vi "rep_cap_compose_cmd.vi"(5 "Repeated Capability":string, 7 "Attribute":T1={"Identifier"="", "Descriptive Name"="", "Data Type"=enum."Integer 32", "Command"="", "Access"=enum."Read/Write", "Range Table"="", "Read Callback"="", "Write Callback"="", "Supported Models"="", "Instrument Options"="", "Index"=0, "OPC Wait"=FALSE, "No Status Check"=FALSE, "Cache Only"=FALSE}, 8 "error in":errorcluster caption="error in (no error)", 11 "VISA resource name":refnum<visa-resource-name>) -> (0 "error out":errorcluster, 2 "Command out":string, 3 "VISA resource name out":refnum<visa-resource-name>)   [LabVIEW 2022 SP3, in "hmp4000_rsidr_core.lvlib"]
uses:
  hmp4000_rsidr_core.lvlib
  type_Attribute.ctl
  type_Attribute_Data_Type.ctl
  type_ReadWriteAccess.ctl
  type_AdditionalFlag_Bits.ctl
  _type_Operation_Fgv_RepCap.ctl
  type_Error_Codes.ctl
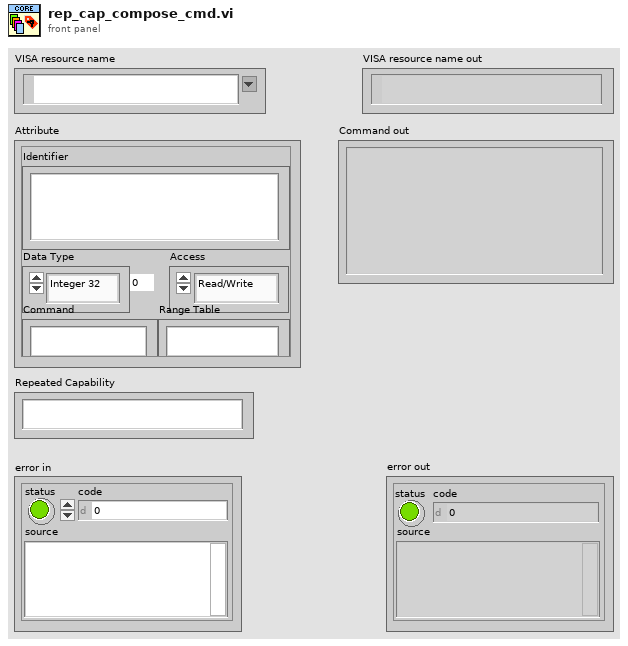
[diagram p1: front panel]
types:
  T1 = typedef "hmp4000_rsidr_core.lvlib/type_Attribute.ctl" = cluster{"Identifier":string, "Descriptive Name":string, "Data Type":T2, "Command":string, "Access":T3, "Range Table":string, "Read Callback":string, "Write Callback":string, "Supported Models":string, "Instrument Options":string, "Index":i32, "OPC Wait":bool, "No Status Check":bool, "Cache Only":bool}
  T2 = typedef "hmp4000_rsidr_core.lvlib/type_Attribute_Data_Type.ctl" = enum16{"Integer 32", "Double", "String", "Boolean", "None", "Integer 64", "RawString"}
  T3 = typedef "hmp4000_rsidr_core.lvlib/type_ReadWriteAccess.ctl" = enum16{"Read Only", "Write Only", "Read/Write"}
  T4 = typedef "hmp4000_rsidr_core.lvlib/type_AdditionalFlag_Bits.ctl" = enum16{"Send LF after Bin Block", "Junk read with io_clear_buffers.vi", "io_clear_buffers: viClear()", "io_clear_buffers: viFlush()", "<NotUsed1>", "Allow Dbl & Int Bin/Ascii read", "*OPC? in check_instrument_error.vi", "<NotUsed2>", "Smart Enum Matching", "Less Strict RepCaps check", "AssureResponseEndWithLF"}
  T5 = typedef "hmp4000_rsidr_core.lvlib/_type_Operation_Fgv_RepCap.ctl" = enum16{"Initialize", "Get Cmd Value", "Reset Rep Cap", "Add Rep Cap", "Remove Rep Cap", "Get Rep Cap ID range", "Get Count", "Clear", "Find Name from NameID", "Get First NameID"}
  T6 = typedef "hmp4000_rsidr_core.lvlib/type_Error_Codes.ctl" = enum16{"No_error", "VISA_err_ResourceNotFound", "VISA_err_Timeout", "VISA_warn_MoreDataAvailable", "RS_err_MissingCallback", "RS_err_InvalidAttribute", "RS_err_InvalidValue", "RS_err_UnknownResource", "RS_err_AlreadyInitialized", "RS_err_InstrumentStatus", "RS_err_BadRepCapName", "RS_err_TypesMismatch", "RS_err_ValueNotSupported", "RS_err_InvalidRngTable", "RS_err_IDqueryFail", "RS_err_UnexpResponse", "VISA_warn_ConfigNotLoaded", "RS_err_AttributeNotReadable", "RS_err_AttributeNotWritable", "RS_err_InstrumentType", "RS_err_InstrumentOption", "VISA_err_InvalidSize", "RS_err_ReliabilityIndicator", "VISA_warn_UnknownStatus", "VISA_warn_TermCharRead", "VISA_err_IO_error", "RS_err_FunctionNotSupported", "VISA_warn_QueueEmpty"}
  T7 = typedef "hmp4000_rsidr_core.lvlib/type_Session_Data.ctl" = cluster{"IDN string":string, "Instrument FW":string, "Instr type":string, "Instr type for err. msg.":string, "Installed Options":string[], "Ignore Error Messages":string, "Logging params":variant, "OPC Timeout":i32, "VISA Timeout":i32, "STB Poll VISA Timeout":i32, "Additional Flags":i32, "Wait Before Read":i32, "Wait Before Write":i32, "Option String Flags":i32, "IO Segment Size":i64, "VISA Access Mode":T8, "Interface Type":T9, "OPC Wait Mode":T10, "Bin Float Number  Format":T11, "Bin Integer Number Format":T12, "Simulate":bool, "VXIcapable":bool, "Duplicate Session":bool, "Add LF to Write":bool, "Logging":bool, "Fast Sweep":bool, "Query Instrument Status":bool, "Check Range":bool, "Check Options":bool}
  T8 = typedef "hmp4000_rsidr_core.lvlib/type_VisaAccessMode.ctl" = u16
  T9 = typedef "hmp4000_rsidr_core.lvlib/type_InterfaceType.ctl" = enum16{"Unknown", "GPIB", "VXI", "GPIB_VXI", "ASRL", "PXI", "TCPIP", "USB", "SOCKET"}
  T10 = typedef "hmp4000_rsidr_core.lvlib/type_OPC_Wait_Mode.ctl" = enum16{"STBpolling", "STBpollingSlow", "STBpollingSuperSlow", "ServiceRequest", "OPCquery"}
  T11 = typedef "hmp4000_rsidr_core.lvlib/type_Binary_Float_Number_Format.ctl" = enum16{"Float_4_Bytes_Swapped", "Float_4_Bytes", "Double_8_Bytes_Swapped", "Double_8_Bytes"}
  T12 = typedef "hmp4000_rsidr_core.lvlib/type_Binary_Integer_Number_Format.ctl" = enum16{"Int32_4_Bytes_Swapped", "Int32_4 Bytes", "Int16_2_Bytes_Swapped", "Int16_2_Bytes"}
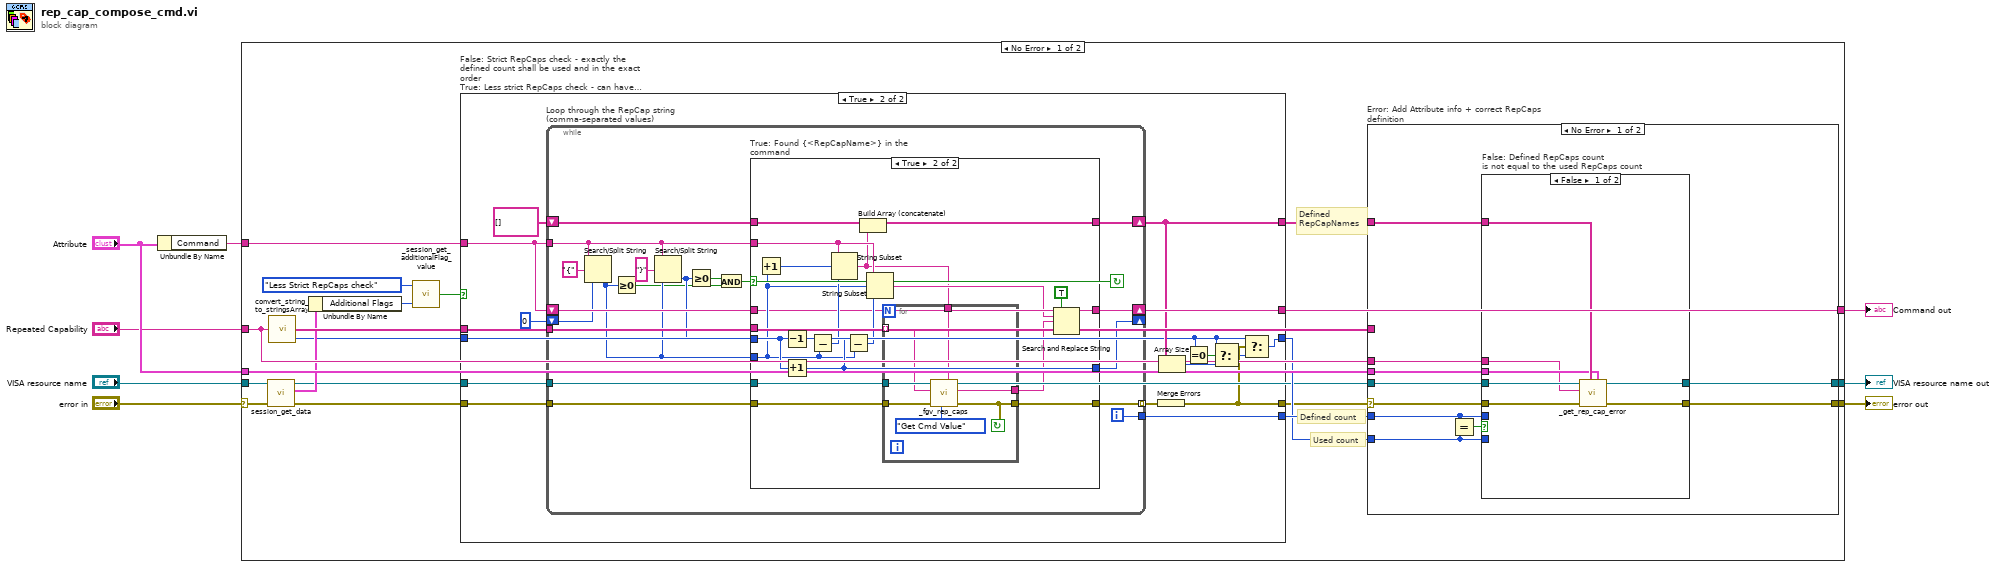
[diagram p0: block diagram]
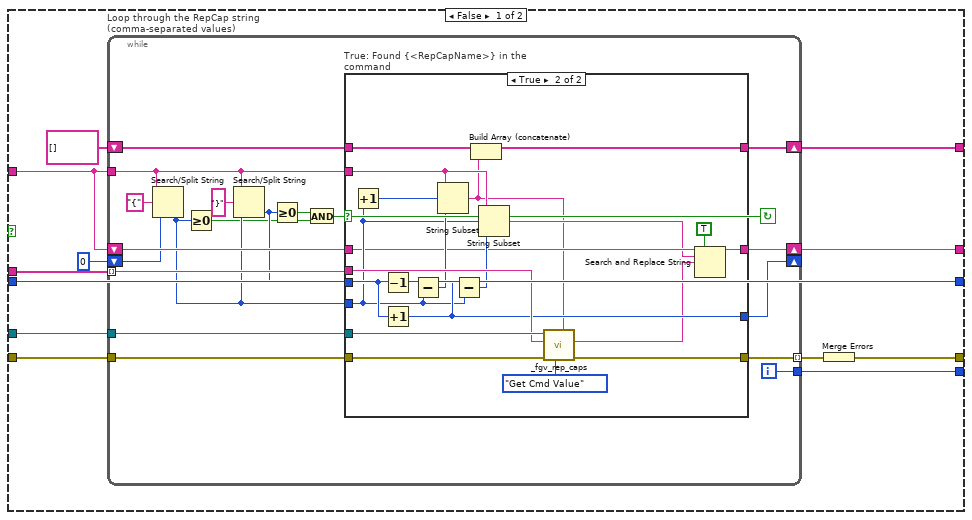
[diagram p2: hidden frame]
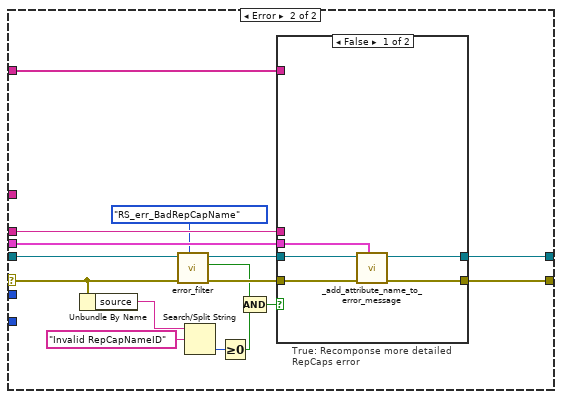
[diagram p6: hidden frame]
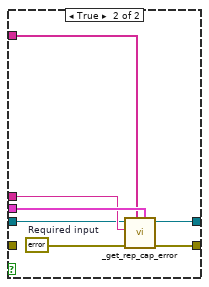
[diagram p7: hidden frame]
diagram:
  n1 = Unbundle By Name("Attribute") -> ("Command"=w1:string)
  n2 = case shown="No Error" "error in" {
    selector: "error in" -> [w19 w198]
    tunnel: "Repeated Capability" -> [w22 _]
    tunnel: [w28 w197] -> w8
    tunnel: [w25 w198] -> w7
    tunnel: w1 -> [w27 w197]
    tunnel: "VISA resource name" -> [w18 w196]
    tunnel: "Attribute" -> [w24 _]
    tunnel: [w21 w196] -> w6
    frame No Error {
      # "Defined count"
      # "Used count"
      # "Defined\nRepCapNames"
      n3 = call "session_get_data.vi"("error in"=w19, "VISA resource name"=w18) -> ("error out"=w17:errorcluster, "Session User Data out"=w16:T7, "VISA resource name out"=w10:refnum<visa-resource-name>)  [unwired: 6 in, 1 out]
      n4 = call "convert_string_to_stringsArray.vi"("String in"=w22) -> ("string array size out"=w13:i32, "string array out"=w20:string[])  [unwired: 3 in]
      n5 = Unbundle By Name(w16) -> ("Additional Flags"=w15:i32)
      n6 = call "_session_get_additionalFlag_value.vi"("AdditionalFlags value in"=w15, "AdditionalFlag bit"=type_AdditionalFlag_Bits."Less Strict RepCaps check") -> ("AdditionalFlag bit value out"=w9:bool)  [unwired: 3 in]
      n7 = case "False: Strict RepCaps check - exactly the defined count shall be used and in the exact order\nTrue: Less strict RepCaps check - can have more repcaps and they can be in random order" shown="True" w9 {
        tunnel: [w40 w99] -> w28
        tunnel: w17 -> [w39 w98]
        tunnel: w27 -> [w38 w97]
        tunnel: [w36 w95] -> w26
        tunnel: [w34 w91] -> w23
        tunnel: [w29 w89] -> w11
        tunnel: w10 -> [w33 w93]
        tunnel: w20 -> [w32 w92]
        tunnel: w13 -> [w31 w85]
        tunnel: [w31 w88] -> w12
        frame False {
          n8 = while "Loop through the RepCap string (comma-separated values)" {
            shift-right: [w59] -> w40
            shift-left: w38 -> [w58]
            tunnel: w33 -> [w56]
            tunnel: w32 -> [w55] mode=indexing
            tunnel: w38 -> [w52]
            shift-right: [w53] -> _
            shift-left: 0 -> [w42]
            tunnel: w39 -> [w57]
            tunnel: [w50] -> w30 mode=indexing
            tunnel: [w45] -> w36
            shift-right: [w43] -> w34
            shift-left: string[] [] -> [w44]
            i -> [w45]
            stop <- w41 continue-if-true
            n9 = Search/Split String(string=w52, search string/char (-)="{", offset (0)=w42) -> (offset of match=w51:i32)  [unwired: 2 out]
            n10 = Greater Or Equal To 0?(x=w51) -> (x >= 0?=w47:bool)
            n11 = Search/Split String(string=w52, search string/char (-)="}", offset (0)=w51) -> (offset of match=w48:i32)  [unwired: 2 out]
            n12 = Greater Or Equal To 0?(x=w48) -> (x >= 0?=w46:bool)
            n13 = And(x=w46, y=w47) -> (x .and. y?=w41:bool)
            n14 = case "True: Found {<RepCapName>} in the command" shown="True" w41 {
              tunnel: w58 -> [w62 w72]
              tunnel: [w62 w70] -> w59
              tunnel: [w61 w71] -> w50
              tunnel: w57 -> [w61 w82]
              tunnel: w56 -> [_ w83]
              tunnel: w55 -> [_ w81]
              tunnel: w48 -> [_ w76]
              tunnel: w51 -> [_ w73]
              tunnel: [_ w75] -> w53
              tunnel: w52 -> [_ w77]
              tunnel: w44 -> [w60 w68]
              tunnel: [w60 w67] -> w43
              frame False {
              }
              frame True {
                n15 = Increment(x=w73) -> (x+1=w80:i32)
                n16 = Decrement(x=w76) -> (x-1=w79:i32)
                n17 = Increment(x=w76) -> (x+1=w75:i32)
                n18 = Subtract(x=w79, y=w73) -> (x-y=w78:i32)
                n19 = String Subset(string=w77, offset (0)=w80, length (rest)=w78) -> (substring=w66:string)
                n20 = Subtract(x=w75, y=w73) -> (x-y=w74:i32)
                n21 = Build Array (concatenate)(w68, w66) -> (w67:string[])
                n22 = String Subset(string=w77, offset (0)=w73, length (rest)=w74) -> (substring=w69:string)
                n23 = call "_fgv_rep_caps.vi"("RepCapName in (\"\")"=w66, "Operation"=_type_Operation_Fgv_RepCap."Get Cmd Value", "error in"=w82, "RepCapNameID in (\"\")"=w81, "VISA resource name"=w83) -> ("error out"=w71:errorcluster, "CmdValue out"=w65:string)  [unwired: 3 in, 2 out]
                n24 = Search and Replace String(replace all?=TRUE ("replace all? (F)"), input string=w72, search string=w69, replace string=w65) -> (result string=w70:string)  [unwired: 4 in, 3 out]
              }
            }
          }
          n25 = Merge Errors(w30) -> (w29:errorcluster)
        }
        frame True {
          n26 = while "Loop through the RepCap string (comma-separated values)" {
            shift-right: [w118] -> w99
            shift-left: w97 -> [w117]
            tunnel: w93 -> [w115]
            tunnel: w92 -> [w114]
            tunnel: w97 -> [w111]
            shift-right: [w112] -> _
            shift-left: 0 -> [w101]
            tunnel: w98 -> [w116]
            tunnel: [w109] -> w90 mode=indexing
            tunnel: [w104] -> w95
            shift-right: [w102] -> w91
            shift-left: string[] [] -> [w103]
            i -> [w104]
            stop <- w100 continue-if-true
            n27 = Search/Split String(string=w111, search string/char (-)="{", offset (0)=w101) -> (offset of match=w110:i32)  [unwired: 2 out]
            n28 = Greater Or Equal To 0?(x=w110) -> (x >= 0?=w106:bool)
            n29 = Search/Split String(string=w111, search string/char (-)="}", offset (0)=w110) -> (offset of match=w107:i32)  [unwired: 2 out]
            n30 = Greater Or Equal To 0?(x=w107) -> (x >= 0?=w105:bool)
            n31 = And(x=w105, y=w106) -> (x .and. y?=w100:bool)
            n32 = case "True: Found {<RepCapName>} in the command" shown="True" w100 {
              tunnel: w117 -> [w121 w131]
              tunnel: [w121 w130] -> w118
              tunnel: [w120 w122] -> w109
              tunnel: w116 -> [w120 w140]
              tunnel: w115 -> [_ w141]
              tunnel: w114 -> [_ w123]
              tunnel: w107 -> [_ w135]
              tunnel: w110 -> [_ w132]
              tunnel: [_ w134] -> w112
              tunnel: w111 -> [_ w136]
              tunnel: w103 -> [w119 w128]
              tunnel: [w119 w127] -> w102
              frame False {
              }
              frame True {
                n33 = Increment(x=w132) -> (x+1=w139:i32)
                n34 = Decrement(x=w135) -> (x-1=w138:i32)
                n35 = Increment(x=w135) -> (x+1=w134:i32)
                n36 = Subtract(x=w138, y=w132) -> (x-y=w137:i32)
                n37 = String Subset(string=w136, offset (0)=w139, length (rest)=w137) -> (substring=w126:string)
                n38 = Subtract(x=w134, y=w132) -> (x-y=w133:i32)
                n39 = Build Array (concatenate)(w128, w126) -> (w127:string[])
                n40 = String Subset(string=w136, offset (0)=w132, length (rest)=w133) -> (substring=w129:string)
                n41 = for {
                  tunnel: w141 -> [w148]
                  tunnel: w140 -> [w147]
                  tunnel: w126 -> [w146]
                  tunnel: [w145] -> w125
                  tunnel: w123 -> [w144] mode=indexing
                  tunnel: [w143] -> w122
                  stop <- w143 continue-if-true
                  n42 = call "_fgv_rep_caps.vi"("RepCapName in (\"\")"=w146, "Operation"=_type_Operation_Fgv_RepCap."Get Cmd Value", "error in"=w147, "RepCapNameID in (\"\")"=w144, "VISA resource name"=w148) -> ("error out"=w143:errorcluster, "CmdValue out"=w145:string)  [unwired: 3 in, 2 out]
                }
                n43 = Search and Replace String(replace all?=TRUE ("replace all? (F)"), input string=w131, search string=w129, replace string=w125) -> (result string=w130:string)  [unwired: 4 in, 3 out]
              }
            }
          }
          n44 = Merge Errors(w90) -> (w89:errorcluster)
          n45 = Array Size(array=w91) -> (size(s)=w84:i32)
          n46 = Equal To 0?(x=w85) -> (x = 0?=w86:bool)
          n47 = Select(t=w85, s=w86, f=w84) -> (s? t:f=w87:i32)
          n48 = Select(t=w85, s=w89, f=w87) -> (s? t:f=w88:i32)
        }
      }
      n49 = case "Error: Add Attribute info + correct RepCaps definition" shown="No Error" w11 {
        selector: w11 -> [w157 w175]
        tunnel: w26 -> [w152 _]
        tunnel: [w156 w181] -> w25
        tunnel: w12 -> [w153 _]
        tunnel: w24 -> [w155 w182]
        tunnel: w22 -> [w154 w180]
        tunnel: w23 -> [w151 w169]
        tunnel: w10 -> [w150 w179]
        tunnel: [w149 w183] -> w21
        tunnel: w20 -> [_ _]
        frame No Error {
          n50 = Equal?(x=w152, y=w153) -> (x = y?=w158:bool)
          n51 = case "False: Defined RepCaps count\nis not equal to the used RepCaps count" shown="False" w158 {
            tunnel: w157 -> [w165 w167]
            tunnel: [w161 w167] -> w156
            tunnel: w155 -> [w160 _]
            tunnel: w154 -> [w159 _]
            tunnel: w153 -> [_ _]
            tunnel: w152 -> [_ _]
            tunnel: w151 -> [w163 _]
            tunnel: w150 -> [w164 w166]
            tunnel: [w162 w166] -> w149
            frame False {
              n52 = call "_get_rep_cap_error.vi"("Attribute"=w160, "Defined RepCapNames in"=w163, "error in"=w165, "Repeated Capability"=w159, "VISA resource name"=w164) -> ("error out"=w161:errorcluster, "VISA resource name out"=w162:refnum<visa-resource-name>)  [unwired: 5 in]
            }
            frame True {
            }
          }
        }
        frame Error {
          n53 = Unbundle By Name(w175) -> ("source"=w168:string)
          n54 = call "error_filter.vi"("Error Enum in"=type_Error_Codes."RS_err_BadRepCapName", "error in"=w175, "VISA resource name"=w179) -> ("error out"=w176:errorcluster, "Code Detected"=w172:bool, "VISA resource name out"=w177:refnum<visa-resource-name>)  [unwired: 6 in]
          n55 = Search/Split String(string=w168, search string/char (-)="Invalid RepCapNameID") -> (offset of match=w174:i32)  [unwired: 1 in, 2 out]
          n56 = Greater Or Equal To 0?(x=w174) -> (x >= 0?=w173:bool)
          n57 = Compound Arithmetic op=AND(w172, w173) -> (w171:bool)
          n58 = case "True: Recomponse more detailed\nRepCaps error" shown="False" w171 {
            tunnel: [w184 w195] -> w183
            tunnel: w182 -> [w186 w194]
            tunnel: [w187 w193] -> w181
            tunnel: w180 -> [_ w192]
            tunnel: w177 -> [w185 w191]
            tunnel: w176 -> [w188 _]
            tunnel: w169 -> [_ w189]
            frame False {
              n59 = call "_add_attribute_name_to_error_message.vi"("Attribute"=w186, "error in"=w188, "VISA resource name"=w185) -> ("error out"=w187:errorcluster, "VISA resource name out"=w184:refnum<visa-resource-name>)  [unwired: 6 in, 1 out]
            }
            frame True {
              w190 = errorcluster {"status"=FALSE, "code"=0, "source"=""}  # Required input
              n60 = call "_get_rep_cap_error.vi"("Attribute"=w194, "Defined RepCapNames in"=w189, "error in"=w190, "Repeated Capability"=w192, "VISA resource name"=w191) -> ("error out"=w193:errorcluster, "VISA resource name out"=w195:refnum<visa-resource-name>)  [unwired: 5 in]
            }
          }
        }
      }
    }
    frame Error {
    }
  }
  "error out" <- w7
  "VISA resource name out" <- w6
  "Command out" <- w8
